vi "Connect.vi"(8 "error in (no error)":errorcluster, 10 "Connection String":string, 11 "MySqlConnection in":refnum<class "DBC.lvclass">) -> (0 "error out":errorcluster, 3 "MySqlConnection out":refnum<class "DBC.lvclass">)   [LabVIEW 2020, in "ORM_DBC_MySql.lvlib" / "DBC.lvclass"]
uses:
  DBC.lvclass
  C:/Program Files/National Instruments/LabVIEW 2020/vi.lib/Viviota/shared/ORM_DBC_dotNet.lvlibp/dbcDotNet/ORM_DBC_dotNet.lvclass
  C:/Program Files/National Instruments/LabVIEW 2020/vi.lib/Viviota/shared/ORM.lvlibp/ORM/DbConnection/DbConnection.lvclass
  C:/Viviota/Projects/R&D/__OpenSource/VIV_ORM/libraries/npgsql/System.Diagnostics.DiagnosticSource.dll
  libraries/npgsql/System.Diagnostics.DiagnosticSource.dll
  C:/Viviota/Projects/R&D/__OpenSource/VIV_ORM/libraries/npgsql/System.Memory.dll
  libraries/npgsql/System.Memory.dll
  C:/Viviota/Projects/R&D/__OpenSource/VIV_ORM/libraries/npgsql/System.Threading.Tasks.Extensions.dll
  libraries/npgsql/System.Threading.Tasks.Extensions.dll
  C:/Viviota/Projects/R&D/__OpenSource/VIV_ORM/libraries/npgsql/Microsoft.Extensions.Logging.Abstractions.dll
  libraries/npgsql/Microsoft.Extensions.Logging.Abstractions.dll
  C:/Viviota/Projects/R&D/__OpenSource/VIV_ORM/libraries/mysql/MySqlConnector.dll
  libraries/mysql/MySqlConnector.dll
  <vilib>/Viviota/shared/ORM_DBC_dotNet.lvlibp/dbcDotNet/Write connection.vi
  <vilib>/Viviota/shared/ORM.lvlibp/ORM/DbConnection/Write ColumnNameEqualsValueFormat.vi
  <vilib>/Viviota/shared/ORM.lvlibp/ORM/DbConnection/Write ColumnNameFormat.vi
  <vilib>/Viviota/shared/ORM.lvlibp/ORM/DbConnection/Write LastIdentityQuery.vi
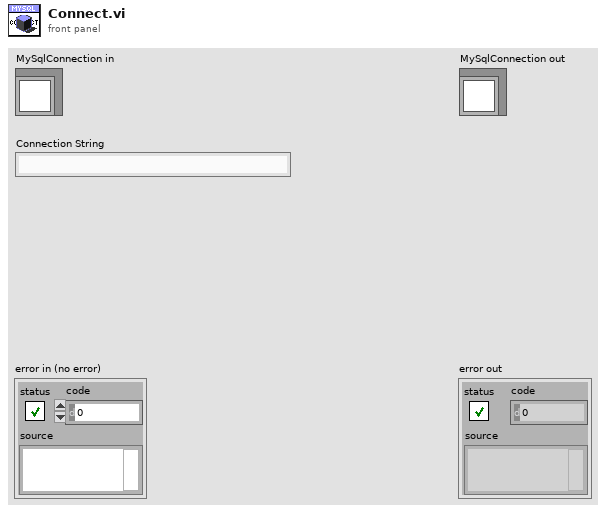
[diagram p1: front panel]
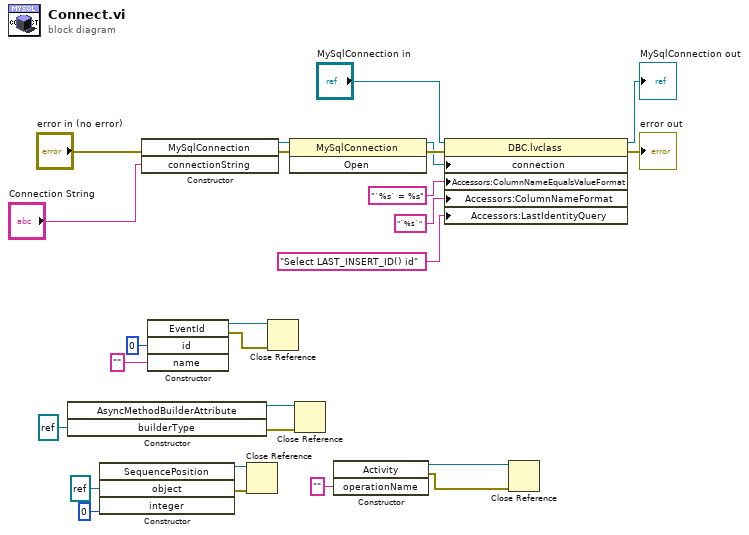
[diagram p0: block diagram]
diagram:
  n1 = constructor class="AsyncMethodBuilderAttribute"("builderType"=refnum<k24> refnum) -> (reference out=w9:refnum<k24>, error out=w10:errorcluster)  [unwired: 3 in, 2 out]
  n2 = constructor class="SequencePosition"("object"=refnum<k24> refnum, "integer"=0) -> (reference out=w6:refnum<k24>, error out=w7:errorcluster)  [unwired: 3 in, 3 out]
  n3 = constructor class="MySqlConnection"(error in="error in (no error)", "connectionString"="Connection String") -> (reference out=w23:refnum<k24>, error out=w24:errorcluster)  [unwired: 2 in, 2 out]
  n4 = constructor class="EventId"("id"=0, "name"="") -> (reference out=w13:refnum<k24>, error out=w14:errorcluster)  [unwired: 3 in, 3 out]
  n5 = Close Reference(reference=w6, error in (no error)=w7) -> ()  [unwired: 1 out]
  n6 = Close Reference(reference=w13, error in (no error)=w14) -> ()  [unwired: 1 out]
  n7 = invoke class="MySqlConnection" method="Open"(reference=w23, error in=w24) -> (reference out=w25:refnum<k24>, error out=w26:errorcluster)  [unwired: 1 in, 1 out]
  n8 = Close Reference(reference=w9, error in (no error)=w10) -> ()  [unwired: 1 out]
  n9 = constructor class="Activity"("operationName"="") -> (reference out=w2:refnum<k24>, error out=w3:errorcluster)  [unwired: 3 in, 2 out]
  n10 = property class="DBC.lvclass"(reference="MySqlConnection in", error in=w26, "connection"=w25, "Accessors:ColumnNameEqualsValueFormat"="`%s` = %s" ("ColumnNameFormat"), "Accessors:ColumnNameFormat"="`%s`" ("ColumnNameFormat"), "Accessors:LastIdentityQuery"="Select LAST_INSERT_ID() id" ("LastIdentityQuery")) -> (reference out=→"MySqlConnection out":refnum<class "DBC.lvclass">, error out=→"error out":errorcluster)
  n11 = Close Reference(reference=w2, error in (no error)=w3) -> ()  [unwired: 1 out]
